vi "pp3_trial_NextState.vi"(8 "Reward CR":bool, 9 "New state countdown (ms)":i64 min=0, 10 "New State":T1=enum."2 (Load Trial)", 11 "State In":T2={"Curr  tr"=0, "Curr (ms)"=0, "Cum (ms)"=0, "Run loop diff"=0, "Tone countdown (ms)"=0, "Countdown (ms)"=0, "Curr State"=enum."0 NULL", "Prev State"=enum."1 Habituation", "Rw"=FALSE, "Sw"=FALSE, "Tone\nGate"=FALSE, "Punish"=FALSE, "Current DAQ DO Int"=0, "Current Loaded Trial"={"Trial Type Number"=1, "Trial Type"=enum."GO", "Trial Weight"=100, "Shock (mA)"=0.3, "Duration (ms)"=0.25, "Sound Type"=enum."04 FM Sweep", "Stim P1"=4000.0, "Stim P2"=0.0, "Stim P3"=0.0, "Stim P4"=2000.0, "DAQ Amplitude (V)"=0.25}, "Next Trial (for display purposes)"={"Trial Type Number"=1, "Trial Type"=enum."GO", "Trial Weight"=100, "Shock (mA)"=0.3, "Duration (ms)"=0.25, "Sound Type"=enum."04 FM Sweep", "Stim P1"=4000.0, "Stim P2"=0.0, "Stim P3"=0.0, "Stim P4"=2000.0, "DAQ Amplitude (V)"=0.25}, "Total trials memo"=0, "State start cum memo (ms)"=0, "Last dur jump time memo (ms)"=0, "Last dur shock time memo (ms)"=0, "Tone repeat memo (ms)"=0, "Webcam on"=FALSE, "Webcam recording"=FALSE, "State update flag"=FALSE, "Last loaded shock voltage"=0.0, "Vid upd"=enum."0"} {"Current DAQ DO Int" format="%016b"; "Next Trial (for display purposes)"."DAQ Amplitude (V)" min=0.0 max=5.0 format="%_4g"; "Next Trial (for display purposes)"."Shock (mA)" min=-1.0 max=5.0; "Next Trial (for display purposes)"."Trial Weight" step=1; "Next Trial (for display purposes)"."Duration (ms)" min=0.0 max=1.0; "Next Trial (for display purposes)"."Trial Type Number" min=1 max=256 step=1; "Current Loaded Trial"."DAQ Amplitude (V)" min=0.0 max=5.0 format="%_4g"; "Current Loaded Trial"."Shock (mA)" min=-1.0 max=5.0; "Current Loaded Trial"."Trial Weight" step=1; "Current Loaded Trial"."Duration (ms)" min=0.0 max=1.0; "Current Loaded Trial"."Trial Type Number" min=1 max=256 step=1}) -> (3 "State Out":T2={"Curr  tr"=0, "Curr (ms)"=0, "Cum (ms)"=0, "Run loop diff"=0, "Tone countdown (ms)"=0, "Countdown (ms)"=0, "Curr State"=enum."0 NULL", "Prev State"=enum."1 Habituation", "Rw"=FALSE, "Sw"=FALSE, "Tone\nGate"=FALSE, "Punish"=FALSE, "Current DAQ DO Int"=0, "Current Loaded Trial"={"Trial Type Number"=1, "Trial Type"=enum."GO", "Trial Weight"=100, "Shock (mA)"=0.3, "Duration (ms)"=0.25, "Sound Type"=enum."04 FM Sweep", "Stim P1"=4000.0, "Stim P2"=0.0, "Stim P3"=0.0, "Stim P4"=2000.0, "DAQ Amplitude (V)"=0.25}, "Next Trial (for display purposes)"={"Trial Type Number"=1, "Trial Type"=enum."GO", "Trial Weight"=100, "Shock (mA)"=0.3, "Duration (ms)"=0.25, "Sound Type"=enum."04 FM Sweep", "Stim P1"=4000.0, "Stim P2"=0.0, "Stim P3"=0.0, "Stim P4"=2000.0, "DAQ Amplitude (V)"=0.25}, "Total trials memo"=0, "State start cum memo (ms)"=0, "Last dur jump time memo (ms)"=0, "Last dur shock time memo (ms)"=0, "Tone repeat memo (ms)"=0, "Webcam on"=FALSE, "Webcam recording"=FALSE, "State update flag"=FALSE, "Last loaded shock voltage"=0.0, "Vid upd"=enum."0"} {"Current DAQ DO Int" format="%016b"; "Next Trial (for display purposes)"."DAQ Amplitude (V)" min=0.0 max=5.0 format="%_4g"; "Next Trial (for display purposes)"."Shock (mA)" min=-1.0 max=5.0; "Next Trial (for display purposes)"."Trial Weight" step=1; "Next Trial (for display purposes)"."Duration (ms)" min=0.0 max=1.0; "Next Trial (for display purposes)"."Trial Type Number" min=1 max=256 step=1; "Current Loaded Trial"."DAQ Amplitude (V)" min=0.0 max=5.0 format="%_4g"; "Current Loaded Trial"."Shock (mA)" min=-1.0 max=5.0; "Current Loaded Trial"."Trial Weight" step=1; "Current Loaded Trial"."Duration (ms)" min=0.0 max=1.0; "Current Loaded Trial"."Trial Type Number" min=1 max=256 step=1})   [LabVIEW 2013]
uses:
  pp3_CTL_StateInfo.ctl
  pp3_CTL_State.ctl
  pp3_CTL_Trial.ctl
  pp3_CTL_TrialType.ctl
  labolabo2/waveforms/WFTypes.ctl
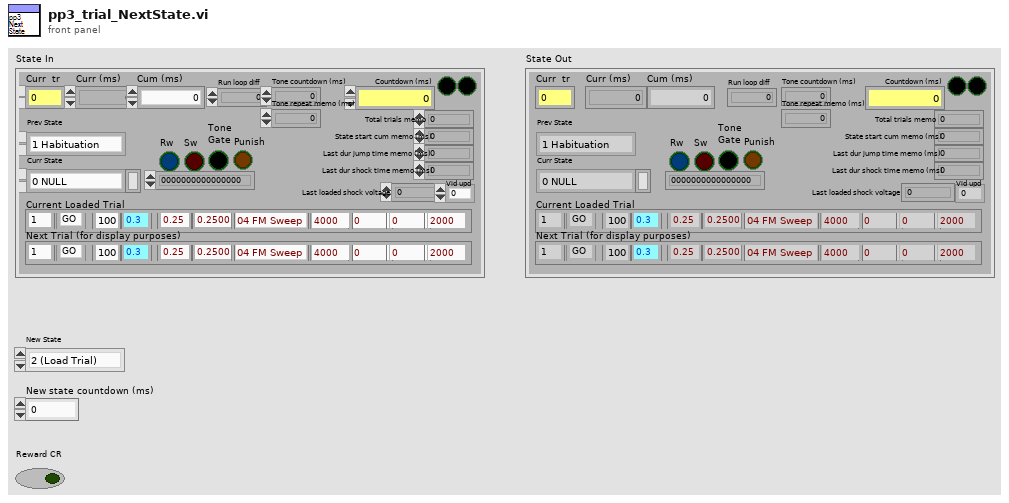
[diagram p1: front panel]
types:
  T1 = typedef "pp3_CTL_State.ctl" = enum8{"0 NULL", "1 Habituation", "2 (Load Trial)", "3 Stay Period", "4 Load Audio/Click Delay", "5 GO Trial", "6 GO Jumped", "7 GO Timeout", "8 NOGO Trial", "9 NOGO Jumped", "10 NOGO Timeout", "11 TEST Trial", "12 TEST Jumped", "13 TEST Timeout", "14 Intertrial Interval", "15 Done"}
  T2 = typedef "pp3_CTL_StateInfo.ctl" = cluster{"Curr  tr":u16, "Curr (ms)":u32, "Cum (ms)":i64, "Run loop diff":i64, "Tone countdown (ms)":i64, "Countdown (ms)":i64, "Curr State":T1, "Prev State":T1, "Rw":bool, "Sw":bool, "Tone\nGate":bool, "Punish":bool, "Current DAQ DO Int":u16, "Current Loaded Trial":T3, "Next Trial (for display purposes)":T3, "Total trials memo":i64, "State start cum memo (ms)":i64, "Last dur jump time memo (ms)":i64, "Last dur shock time memo (ms)":i64, "Tone repeat memo (ms)":i64, "Webcam on":bool, "Webcam recording":bool, "State update flag":bool, "Last loaded shock voltage":dbl, "Vid upd":enum16{"0", "1", "2", "3", "4", "5", "6", "7", "8", "9"}}
  T3 = typedef "pp3_CTL_Trial.ctl" = cluster{"Trial Type Number":i16, "Trial Type":T4, "Trial Weight":u32, "Shock (mA)":dbl, "Duration (ms)":dbl, "Sound Type":T5, "Stim P1":dbl, "Stim P2":dbl, "Stim P3":dbl, "Stim P4":dbl, "DAQ Amplitude (V)":dbl}
  T4 = typedef "pp3_CTL_TrialType.ctl" = enum16{"OFF", "GO", "NOGO", "TEST"}
  T5 = typedef "WFTypes.ctl" = enum16{"00 NULL", "01 DC", "02 Noise", "03 Pure Tone", "04 FM Sweep"}
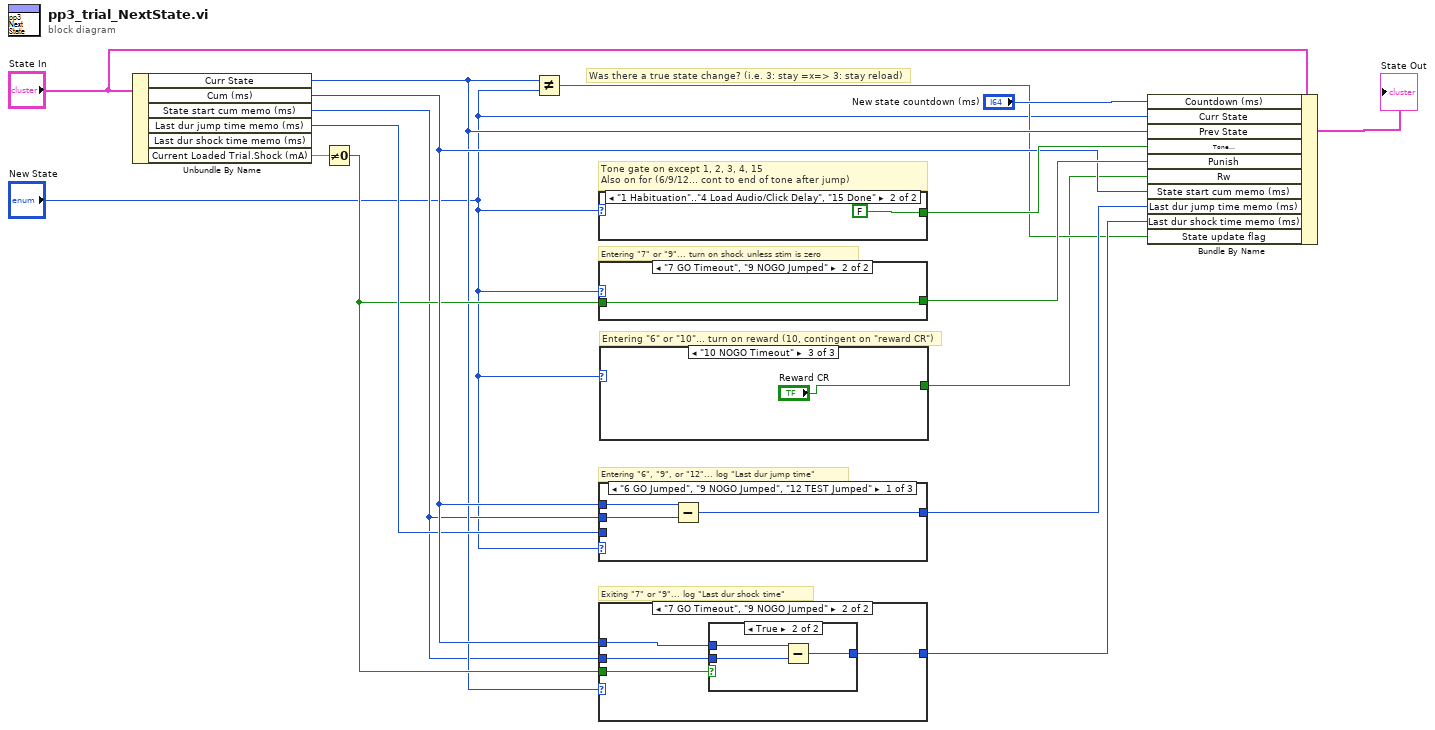
[diagram p0: block diagram]
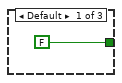
[diagram p2: hidden frame]
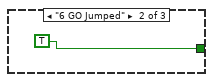
[diagram p3: hidden frame]
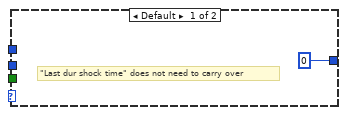
[diagram p4: hidden frame]
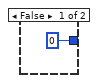
[diagram p5: hidden frame]
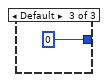
[diagram p7: hidden frame]
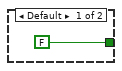
[diagram p8: hidden frame]
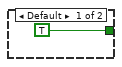
[diagram p9: hidden frame]
diagram:
  # "Entering \"6\" or \"10\"... turn on reward (10, contingent on \"reward CR\")"
  # "Was there a true state change? (i.e. 3: stay =x=> 3: stay reload)"
  # "Entering \"7\" or \"9\"... turn on shock unless stim is zero"
  # "Entering \"6\", \"9\", or \"12\"... log \"Last dur jump time\""
  # "Tone gate on except 1, 2, 3, 4, 15\nAlso on for (6/9/12... cont to end of tone after jump)"
  # "Exiting \"7\" or \"9\"... log \"Last dur shock time\""
  n1 = Unbundle By Name("State In") -> ("Curr State"=w5:T1, "Cum (ms)"=w11:i64, "State start cum memo (ms)"=w3:i64, "Last dur jump time memo (ms)"=w10:i64, "Current Loaded Trial.Shock (mA)"=w7:dbl)  [unwired: 1 out]
  n2 = Not Equal To 0?(x=w7) -> (x != 0?=w6:bool)
  n3 = Not Equal?(x=w5, y="New State") -> (x != y?=w4:bool)
  n4 = case shown="\"1 Habituation\"..\"4 Load Audio/Click Delay\", \"15 Done\"" "New State" {
    tunnel: [TRUE FALSE] -> w14
    frame Default {
    }
    frame "1 Habituation".."4 Load Audio/Click Delay", "15 Done" {
    }
  }
  n5 = case shown="\"7 GO Timeout\", \"9 NOGO Jumped\"" "New State" {
    tunnel: [FALSE w20] -> w13
    tunnel: w6 -> [_ w20]
    frame Default {
    }
    frame "7 GO Timeout", "9 NOGO Jumped" {
    }
  }
  n6 = case shown="\"6 GO Jumped\", \"9 NOGO Jumped\", \"12 TEST Jumped\"" "New State" {
    tunnel: w3 -> [w22 _ _]
    tunnel: w11 -> [w23 _ _]
    tunnel: w10 -> [_ w24 _]
    tunnel: [w21 w24 i64 0 ("Last dur jump time memo (ms)")] -> w12
    frame "6 GO Jumped", "9 NOGO Jumped", "12 TEST Jumped" {
      n7 = Subtract(x=w23, y=w22) -> (x-y=w21:i64)
    }
    frame "14 Intertrial Interval" {
      # "Carry over value if entering \"14: Intertrial Interval\""
    }
    frame Default {
    }
  }
  n8 = case shown="\"7 GO Timeout\", \"9 NOGO Jumped\"" w5 {
    tunnel: w11 -> [_ w30]
    tunnel: [i64 0 ("Last dur shock time memo (ms)") w29] -> w9
    tunnel: w6 -> [_ w28]
    tunnel: w3 -> [_ w27]
    frame Default {
      # "\"Last dur shock time\" does not need to carry over"
    }
    frame "7 GO Timeout", "9 NOGO Jumped" {
      n9 = case shown="True" w28 {
        tunnel: w30 -> [_ w34]
        tunnel: [i64 0 w33] -> w29
        tunnel: w27 -> [_ w32]
        frame False {
        }
        frame True {
          n10 = Subtract(x=w34, y=w32) -> (x-y=w33:i64)
        }
      }
    }
  }
  n11 = case shown="\"10 NOGO Timeout\"" "New State" {
    tunnel: [FALSE TRUE "Reward CR"] -> w1
    frame Default {
    }
    frame "6 GO Jumped" {
    }
    frame "10 NOGO Timeout" {
    }
  }
  n12 = Bundle By Name(cluster="State In", "Countdown (ms)"="New state countdown (ms)", "Curr State"="New State", "Prev State"=w5, "Tone\nGate"=w14, "Punish"=w13, "Rw"=w1, "State start cum memo (ms)"=w11, "Last dur jump time memo (ms)"=w12, "Last dur shock time memo (ms)"=w9, "State update flag"=w4) -> (→"State Out":T2)
